vi "Evaluate Default Trigger.vi"(8 "error in (no error)":errorcluster, 10 "Trigger Data":dbl[](array[numeric]), 11 "Default Trigger in":refnum<class "Default Trigger.lvclass">) -> (0 "error out":errorcluster, 2 "Trigger":bool, 3 "Default Trigger out":refnum<class "Default Trigger.lvclass">)   [LabVIEW 2015, in "Waveform Data Logger Engine.lvlib" / "Default Trigger.lvclass"]
doc: "Evaluates the trigger data and returns whether the specified trigger condition was met."
uses:
  Default Trigger.lvclass
  Default Trigger.lvclass/Default Trigger.ctl
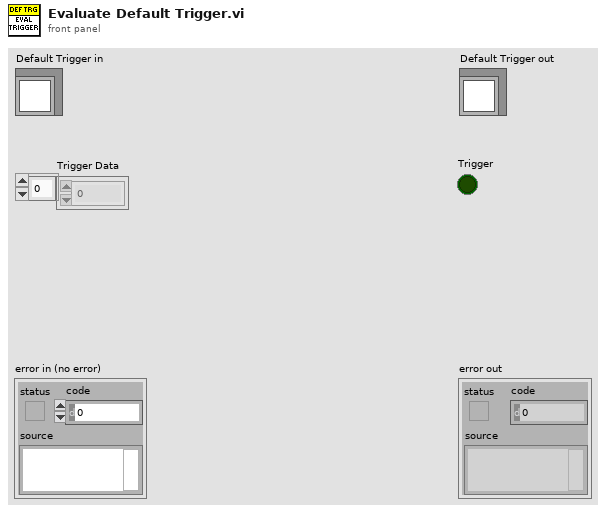
[diagram p1: front panel]
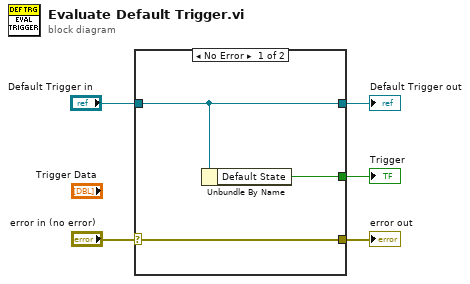
[diagram p0: block diagram]
diagram:
  n1 = case shown="No Error" "error in (no error)" {
    selector: "error in (no error)" -> [w6 w9]
    tunnel: "Default Trigger in" -> [w7 w10]
    tunnel: [w8 _] -> w4
    tunnel: [w7 w10] -> w2
    tunnel: [w6 w9] -> w1
    frame No Error {
      n2 = Unbundle By Name(w7) -> ("Default State"=w8:bool)
    }
    frame Error {
    }
  }
  "error out" <- w1
  "Default Trigger out" <- w2
  "Trigger" <- w4
